vi "Set Max AC voltage.vi"(7 "error in":errorcluster {"code" format="%.0x"}, 9 "Assign  averexp according to the chart on the right":dbl=1.0, 10 "VISA resource name":refnum<visa-resource-name>="GPIB12::28::INSTR") -> (0 "error out":errorcluster {"code" format="%.0x"}, 1 "Read out result":string="UC= 9456.092   PF L= 658.76     NS V=0.10   V\r\n", 2 "Send string":string="UNITS 1;\nSHOW UN", 3 "VISA resource name out":refnum<visa-resource-name>)   [LabVIEW 2016, in "AH2500A.lvclass"]
uses:
  AH2500A.lvclass
panel:
  in  "byte count":u32=128
  # "Set the highest AC voltage limit"
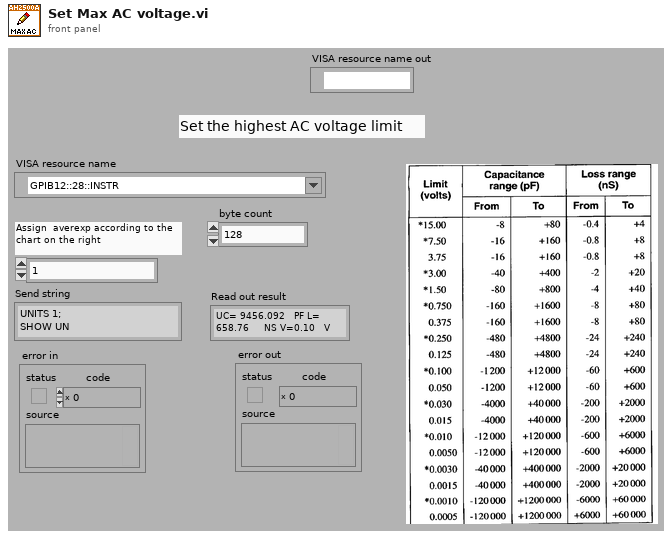
[diagram p1: front panel]
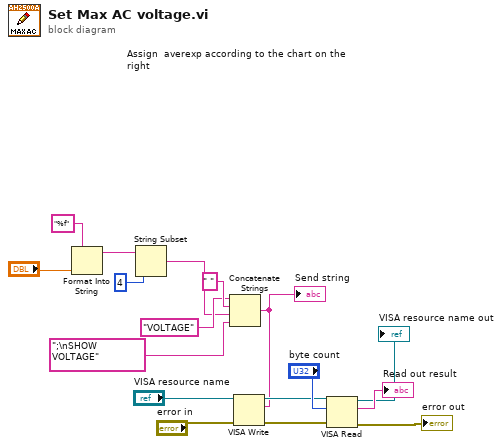
[diagram p0: block diagram]
diagram:
  n1 = Format Into String(format string="%f", "Assign  averexp according to the chart on the right") -> (resulting string=w5:string)  [unwired: 2 in, 1 out]
  n2 = String Subset(string=w5, length (rest)=4 ("length (rest)")) -> (substring=w3:string)  [unwired: 1 in]
  n3 = Concatenate Strings("VOLTAGE" ("string"), " " ("string"), w3, ";\nSHOW VOLTAGE" ("format string")) -> (w8:string)
  "Send string" <- w8
  n4 = VISA Write(VISA resource name="VISA resource name", write buffer=w8, error in (no error)="error in") -> (VISA resource name out=w11:refnum<visa-resource-name>, error out=w10:errorcluster)  [unwired: 1 out]
  n5 = VISA Read(VISA resource name=w11, byte count="byte count", error in (no error)=w10) -> (VISA resource name out=→"VISA resource name out":refnum<visa-resource-name>, read buffer=→"Read out result":string, error out=→"error out":errorcluster)  [unwired: 1 out]
